vi "PID Calibrator main.vi"() -> ()   [LabVIEW 2022 SP3]
uses:
  <vilib>/Instr/_visa.llb/VISA Configure Serial Port (Instr).vi
panel:
  in  "VISA resource name":refnum<visa-resource-name>
  in  "stop":bool
  out "Position":u32(graph)
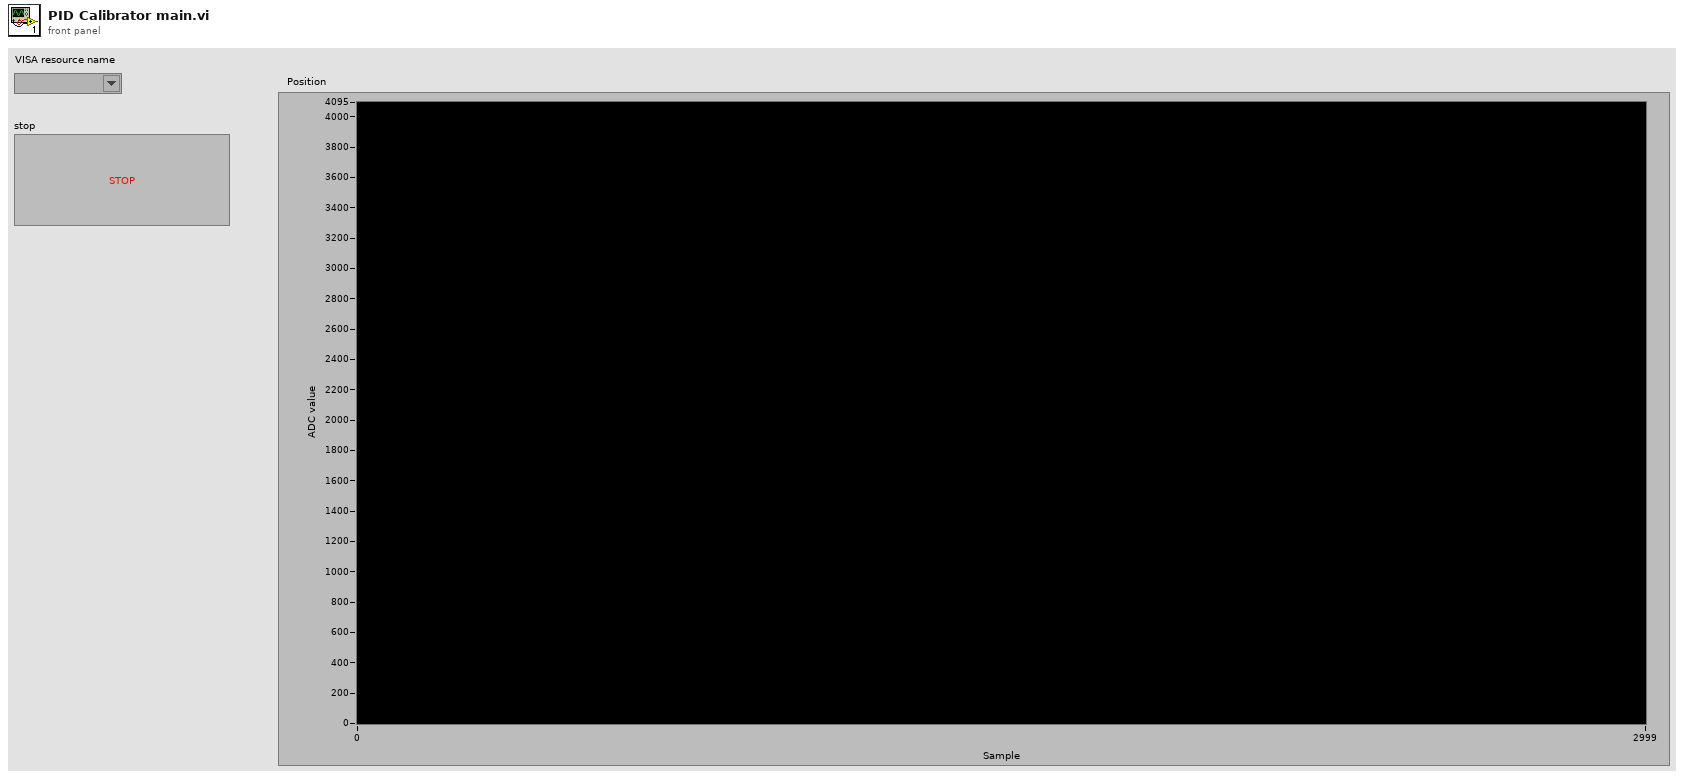
[diagram p1: front panel]
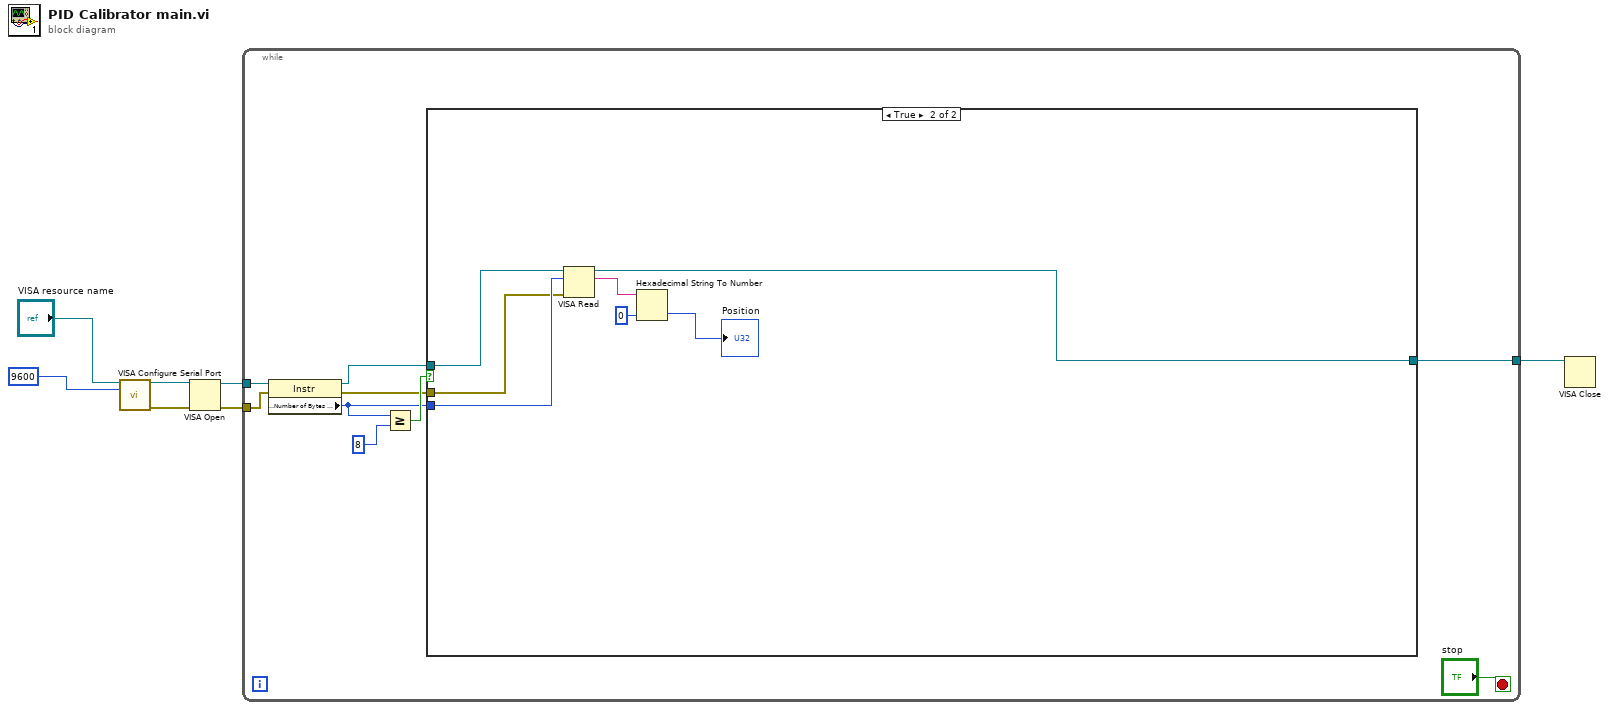
[diagram p0: block diagram]
diagram:
  n1 = call-poly "VISA Configure Serial Port"("VISA resource name"="VISA resource name", "baud rate (9600)"=u32 9600) -> ("VISA resource name out"=w6:refnum<visa-resource-name>, "error out"=w3:errorcluster)  [unwired: 12 in]
  n2 = VISA Open(error in (no error)=w3, VISA resource name=w6) -> (VISA resource name=w5:refnum<visa-resource-name>, error out=w2:errorcluster)  [unwired: 3 in]
  n3 = while {
    tunnel: w5 -> [w16]
    tunnel: [w8] -> w4
    tunnel: w2 -> [w10]
    stop <- "stop" stop-if-true
    n4 = property class="Instr"(reference=w16, error in=w10) -> (reference out=w12:refnum<visa-resource-name>, error out=w9:errorcluster, "Serial Settings:Number of Bytes at Serial Port"=w11:u32)
    n5 = Greater Or Equal?(x=w11, y=u32 8) -> (x >= y?=w13:bool)
    n6 = case shown="True" w13 {
      tunnel: w12 -> [w17 w24]
      tunnel: w11 -> [_ w23]
      tunnel: w9 -> [_ w22]
      tunnel: [w17 w18] -> w8
      frame False {
      }
      frame True {
        n7 = VISA Read(VISA resource name=w24, byte count=w23, error in (no error)=w22) -> (VISA resource name out=w18:refnum<visa-resource-name>, read buffer=w21:string)  [unwired: 2 out]
        n8 = Hexadecimal String To Number(string=w21, default (0uL)=u32 0 ("default (0 U32)")) -> (number=→"Position":u32)  [unwired: 1 in, 1 out]
      }
    }
  }
  n9 = VISA Close(VISA resource name=w4) -> ()  [unwired: 1 in, 1 out]
